vi "SetData.vi"(8 "error in (no error)":errorcluster caption="Fehler (Eingang, kein Fehler)", 9 "Data":variant, 10 "Key":string, 11 "Dictionary Eingang":refnum<class "Dictionary.lvclass"> caption="DNL_LabVIEW Object in") -> (0 "error out":errorcluster caption="Fehler (Ausgang)", 3 "Dictionary Ausgang":refnum<class "Dictionary.lvclass"> caption="DNL_LabVIEW Object out")   [LabVIEW 2013, in "LvDictionary.lvlib" / "Dictionary.lvclass"]
uses:
  Dictionary.lvclass
  Dictionary.lvclass/Dictionary.ctl
  Properties/GetDict.vi
  Properties/SetDict.vi
  <vilib>/Utility/error.llb/Error Cluster From Error Code.vi
  <vilib>/ErrorRing/Error Ring.xnode
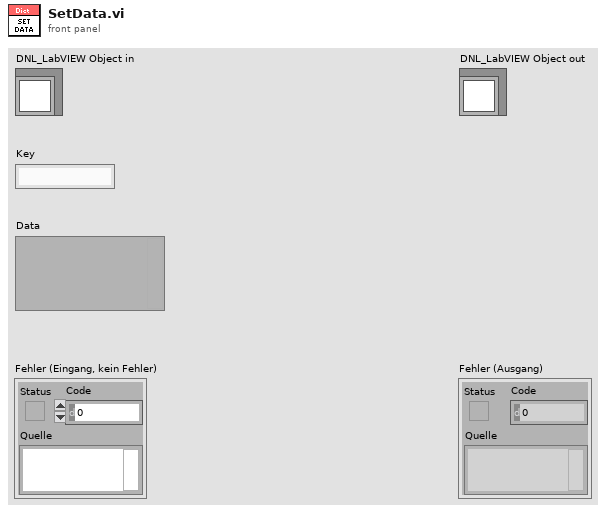
[diagram p1: front panel]
types:
  T1 = cluster{"status":bool, "code":bool, "source":bool}
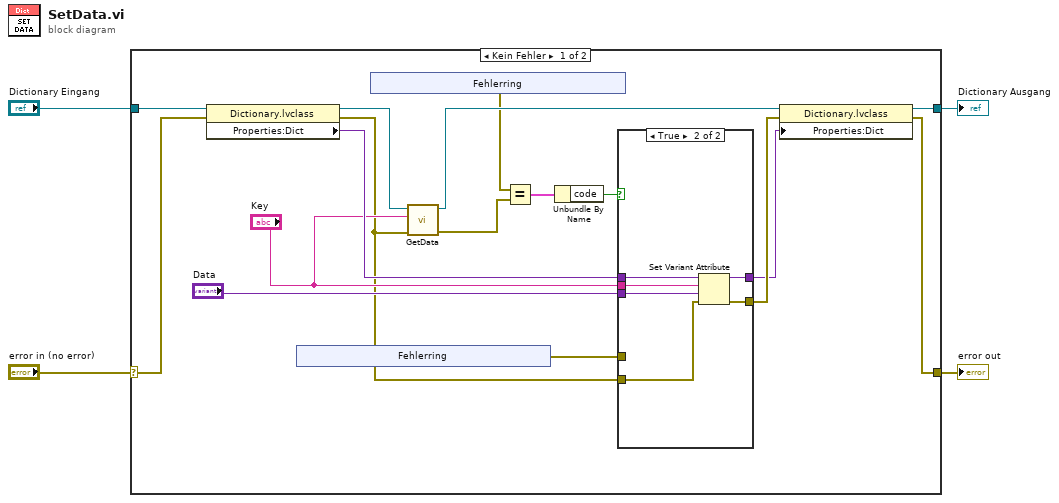
[diagram p0: block diagram]
diagram:
  n1 = case shown="Kein Fehler" "error in (no error)" {
    selector: "error in (no error)" -> [w14 w41]
    tunnel: [w19 w41] -> w3
    tunnel: [w20 w40] -> w1
    tunnel: "Dictionary Eingang" -> [w21 w40]
    frame No Error {
      n2 = property class="Dictionary.lvclass"(reference=w21, error in=w14) -> (reference out=w13:refnum<class "Dictionary.lvclass">, error out=w10:errorcluster, "Properties:Dict"=w16:variant)
      n3 = xnode ("Fehlerring")() -> ("Fehler (Ausgang)"=w9:errorcluster)
      n4 = xnode "Fehlerring"() -> ("Fehler (Ausgang)"=w8:errorcluster)
      n5 = call-dynamic "GetData.vi"("error in (no error)"=w10, "Name"="Key", "Dictionary Eingang"=w13) -> ("error out"=w7:errorcluster, "Dictionary Ausgang"=w11:refnum<class "Dictionary.lvclass">)  [unwired: 6 in, 1 out]
      n6 = Equal?(x=w8, y=w7) -> (x = y?=w6:T1)
      n7 = Unbundle By Name(w6) -> ("code"=w5:bool)
      n8 = case shown="True" w5 {
        tunnel: [w32 w39] -> w18
        tunnel: [w33 w38] -> w17
        tunnel: w16 -> [w33 w37]
        tunnel: "Data" -> [_ w36]
        tunnel: "Key" -> [_ w35]
        tunnel: w10 -> [_ w34]
        tunnel: w9 -> [w32 _]
        frame False {
        }
        frame True {
          n9 = Set Variant Attribute(Variant=w37, name=w35, value=w36, error in=w34) -> (Variant out=w38:variant, error out=w39:errorcluster)  [unwired: 1 out]
        }
      }
      n10 = property class="Dictionary.lvclass"(reference=w11, error in=w18, "Properties:Dict"=w17) -> (reference out=w20:refnum<class "Dictionary.lvclass">, error out=w19:errorcluster)
    }
    frame Error {
    }
  }
  "error out" <- w3
  "Dictionary Ausgang" <- w1
